vi "Variant to Class.vi"(8 "error in (no error)":errorcluster, 10 "Data in":variant, 11 "Serializable Node in":refnum<class "Serializable Node.lvclass">) -> (0 "error out":errorcluster, 2 "Data Out":variant, 3 "Serializable Node out":refnum<class "Serializable Node.lvclass">)   [LabVIEW 2014, in "Serializable Node.lvclass"]
uses:
  Serializable Node.lvclass
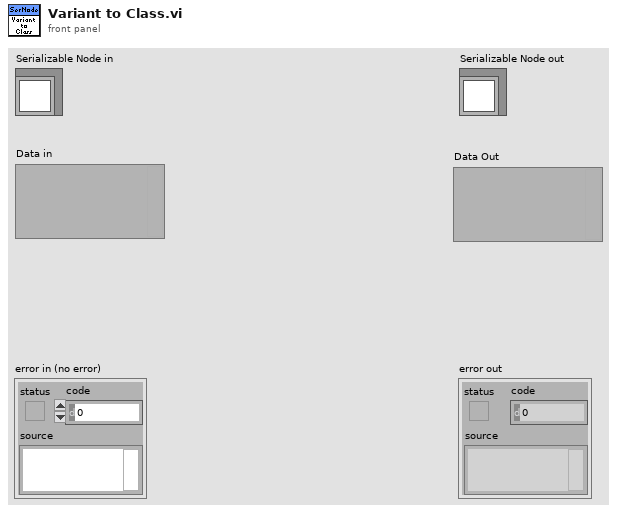
[diagram p1: front panel]
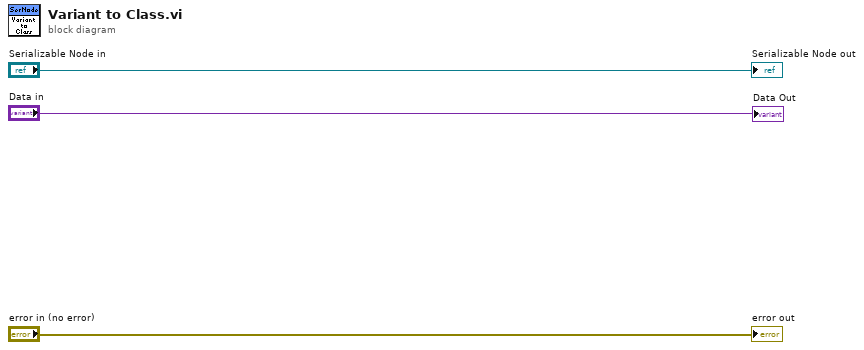
[diagram p0: block diagram]
diagram:
  "error out" <- "error in (no error)"
  "Serializable Node out" <- "Serializable Node in"
  "Data Out" <- "Data in"
